vi "LP RT Streamer State Decide for status.vi"(8 "error in (no error)":errorcluster, 10 "RefreshRate":i32, 11 "Queue in":refnum<queue>) -> (0 "error out":errorcluster, 1 "Data":variant, 2 "CMD":T1, 3 "queue out":refnum<queue>)   [LabVIEW 2015]
uses:
  Controls/RT Streamer State.ctl
  Controls/RT Streamer Queue element.ctl
  Controls/Log Thread Name.ctl
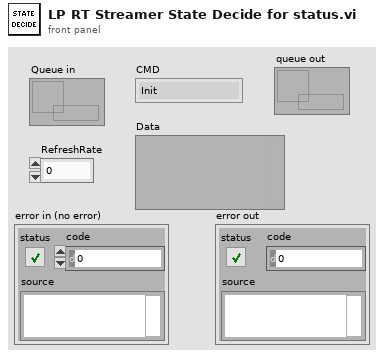
[diagram p1: front panel]
types:
  T1 = typedef "RT Streamer State.ctl" = enum16{"Init", "Idle", "Stream", "Listen", "SetRefrashRate", "SendCmdAck", "SendCmdDone", "SendSysState", "StartRecord", "Green Cordinates", "Error"}
  T2 = typedef "RT Streamer Queue element.ctl" = cluster{"CMD":T1, "Data":variant, "Error in":errorcluster}
  T3 = typedef "Log Thread Name.ctl" = enum16{"Motor R", "Generic", "Motor P", "Motor Y", "StreamClient", "Stream Server", "Sequencer"}
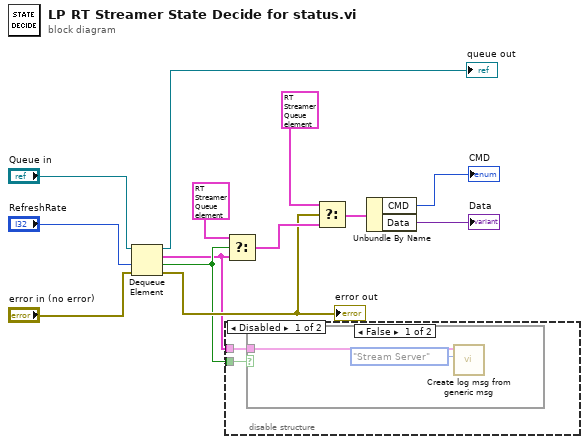
[diagram p0: block diagram]
diagram:
  n1 = Dequeue Element(queue="Queue in", timeout in ms (-1)="RefreshRate", error in (no error)="error in (no error)") -> (queue out=→"queue out":refnum<queue>, element=w1:T2, timed out?=w2:bool, error out=w3:errorcluster)
  "error out" <- w3
  n2 = disable-structure shown="Disabled" {
    disable-tunnel: w2 -> [w15 _]
    disable-tunnel: w1 -> [w14 _]
    frame Disabled {
      n3 = case shown="False" w15 {
        tunnel: w14 -> [w16 _]
        frame False {
          n4 = call "Create log msg from generic msg.vi"("Thread"=Log_Thread_Name."Stream Server", "variant"=w16) -> ()  [unwired: 10 in]
        }
        frame True {
        }
      }
    }
    frame Enabled {
    }
  }
  n5 = Select(t=T2 {"CMD"=enum."SendSysState", "Data"=variant, "Error in"={"status"=FALSE, "code"=0, "source"=""}}, s=w2, f=w1) -> (s? t:f=w7:T2)
  n6 = Select(t=T2 {"CMD"=enum."Error", "Data"=variant, "Error in"={"status"=FALSE, "code"=0, "source"=""}}, s=w3, f=w7) -> (s? t:f=w9:T2)
  n7 = Unbundle By Name(w9) -> ("CMD"=→"CMD":T1, "Data"=→"Data":variant)
